vi "Conversion Factor.vi"(8 "error in (no error)":errorcluster, 10 "Unit":string) -> (0 "error out":errorcluster, 2 "Conversion factor":dbl)   [LabVIEW 2019]
doc: "This VI returns the conversion factor to turn a unit with a prefix to it's base unit.\nRecognized units: A, O, Ohm, RATIO, V, Vpp, dB, dBm \nRecognized prefixes: G, M, k, m, u, n, p"
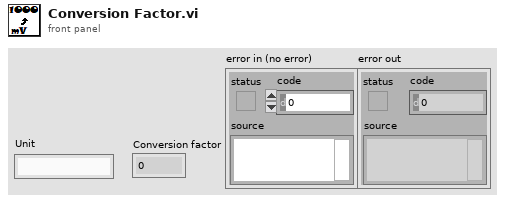
[diagram p1: front panel]
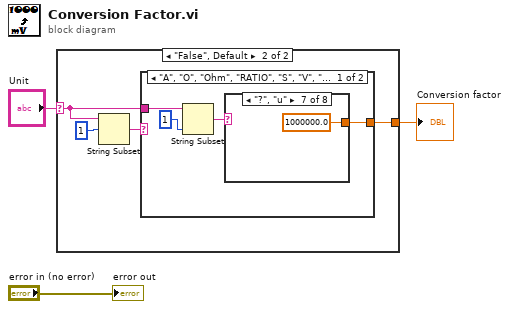
[diagram p0: block diagram]
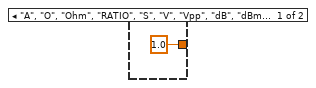
[diagram p2: hidden frame]
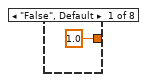
[diagram p3: hidden frame]
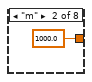
[diagram p4: hidden frame]
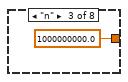
[diagram p5: hidden frame]
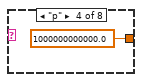
[diagram p6: hidden frame]
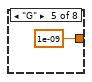
[diagram p7: hidden frame]
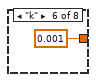
[diagram p8: hidden frame]
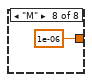
[diagram p9: hidden frame]
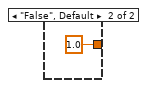
[diagram p10: hidden frame]
diagram:
  n1 = case shown="\"False\", Default" "Unit" {
    selector: "Unit" -> [_ w5]
    tunnel: [1.0 w7] -> w2
    frame "A", "O", "Ohm", "RATIO", "S", "V", "Vpp", "dB", "dBm", "s" {
    }
    frame "False", Default {
      n2 = String Subset(string=w5, offset (0)=1) -> (substring=w6:string)  [unwired: 1 in]
      n3 = case shown="\"A\", \"O\", \"Ohm\", \"RATIO\", \"S\", \"V\", \"Vpp\", \"dB\", \"dBm\", \"s\"" w6 {
        tunnel: [w10 1.0] -> w7
        tunnel: w5 -> [w9 _]
        frame "A", "O", "Ohm", "RATIO", "S", "V", "Vpp", "dB", "dBm", "s" {
          n4 = String Subset(string=w9, length (rest)=1 ("length (rest)")) -> (substring=w11:string)  [unwired: 1 in]
          n5 = case shown="\"?\", \"u\"" w11 {
            tunnel: [1.0 1000.0 1000000000.0 1000000000000.0 1e-09 0.001 1000000.0 1e-06] -> w10
            frame "False", Default {
            }
            frame "m" {
            }
            frame "n" {
            }
            frame "p" {
            }
            frame "G" {
            }
            frame "k" {
            }
            frame "?", "u" {
            }
            frame "M" {
            }
          }
        }
        frame "False", Default {
        }
      }
    }
  }
  "Conversion factor" <- w2
  "error out" <- "error in (no error)"
